vi "Collection.vi"(8 "error in (no error)":errorcluster, 10 "Array":refnum<class "Readable.lvclass">[](array[class]), 11 "Collection.lvclass in":refnum<class "Collection.lvclass">) -> (0 "error out":errorcluster, 3 "Collection.lvclass out":refnum<class "Collection.lvclass">)   [LabVIEW 2012, in "Collection.lvclass"]
uses:
  Collection.lvclass
  Readable/Readable.lvclass
  Readable/Channel Units.ctl
  Collection.lvclass/Collection.ctl
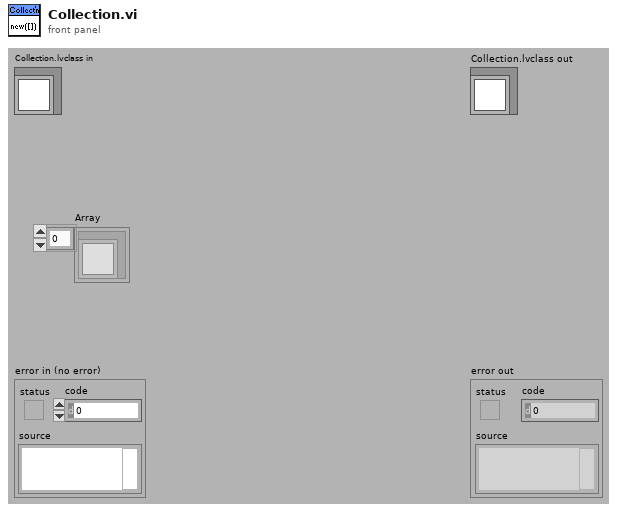
[diagram p1: front panel]
types:
  T1 = typedef "Readable.lvclass/Channel Units.ctl" = string[]
  T2 = typedef "Readable.lvclass/Channel Names.ctl" = string[]
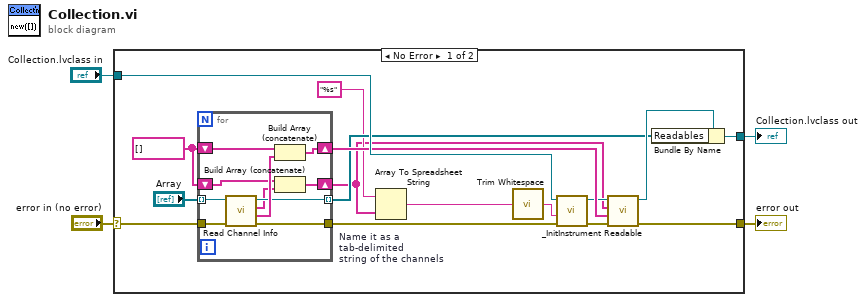
[diagram p0: block diagram]
diagram:
  n1 = case shown="No Error" "error in (no error)" {
    selector: "error in (no error)" -> [w14 w31]
    tunnel: [w13 w31] -> w3
    tunnel: [w20 w32] -> w1
    tunnel: "Collection.lvclass in" -> [w19 w32]
    frame No Error {
      w15 = T1 [] ("Channel Units")
      n2 = for {
        tunnel: "Array" -> [w30] mode=indexing
        shift-right: [w29] -> w16
        shift-left: w15 -> [w27]
        shift-right: [w26] -> w6
        shift-left: w15 -> [w24]
        tunnel: [w25] -> w12 mode=indexing
        tunnel: w14 -> [w23]
        tunnel: [w22] -> w9
        n3 = call "Read Channel Info.vi"("error in (no error)"=w23, "Readable.lvclass in"=w30) -> ("error out"=w22:errorcluster, "Channel Units"=w28:T1, "Channel Names"=w21:T2, "Readable.lvclass out"=w25:refnum<class "Readable.lvclass">)  [unwired: 5 in, 1 out]
        n4 = Build Array (concatenate)(w27, w28) -> (w29:T1)
        n5 = Build Array (concatenate)(w24, w21) -> (w26:T2)
      }
      n6 = Array To Spreadsheet String "Name it as a tab-delimited\nstring of the channels"(array=w6, 3:"%s" ("format string")) -> (spreadsheet string=w7:string)  [unwired: 1 in]
      n7 = call <vilib>:"Trim Whitespace.vi"("string"=w7) -> ("trimmed string"=w5:string)  [unwired: 1 in]
      n8 = call-dynamic "_InitInstrument.vi"("error in (no error)"=w9, "Name"=w5, "Instrument in"=w19) -> ("error out"=w10:errorcluster, "Instrument out"=w11:refnum<class "Collection.lvclass">)  [unwired: 7 in]
      n9 = call "Readable.vi"("error in (no error)"=w10, "Channel Units"=w16, "Channel Names"=w6, "Readable in"=w11) -> ("error out"=w13:errorcluster, "Readable out"=w18:refnum<class "Collection.lvclass">)  [unwired: 6 in]
      n10 = Bundle By Name(cluster=w18, "Readables"=w12) -> (w20:refnum<class "Collection.lvclass">)
    }
    frame Error {
    }
  }
  "error out" <- w3
  "Collection.lvclass out" <- w1
